vi "Select Worksheet by Name.vi"(2 "error in (no error)":errorcluster, 3 "Worksheet Name":string, 4 "Report Ref In":T1) -> (0 "error out":errorcluster, 1 "Report Ref Out":T1)   [LabVIEW 2013, in "XCel Report Engine.lvlib"]
doc: "Selects a worksheet by name and makes it the active worksheet for subsequent report operations.\n\nThe worksheet name must exactly match an existing worksheet in the open workbook. Worksheet name matching is case-sensitive.\n\nAn error is returned if the name is empty or the worksheet does not exist."
uses:
  XCel Report Engine.lvlib
  C:/Users/m.santucci/Documents/ChatGPT/LV_REPORT_ENGINE/LV/DotNet/XCelReportEngine.dll
  LV/DotNet/XCelReportEngine.dll
  Controls/Report Ref.ctl
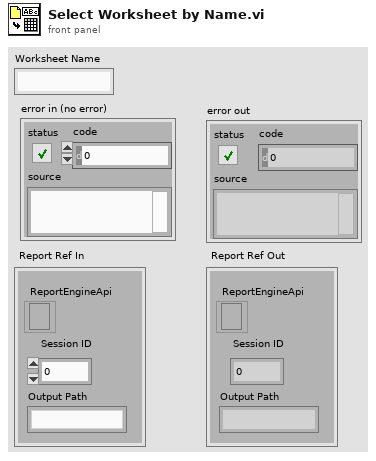
[diagram p1: front panel]
types:
  T1 = typedef "XCel Report Engine.lvlib/Report Ref.ctl" = cluster{"Session ID":i32, "Output Path":string, "ReportEngineApi":refnum<k24>}
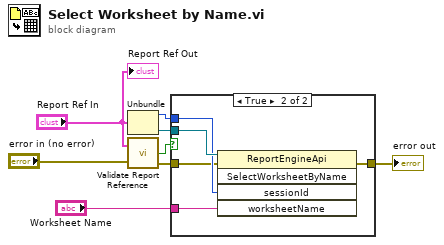
[diagram p0: block diagram]
diagram:
  n1 = Unbundle("Report Ref In") -> ("Session ID"=w7:i32, "ReportEngineApi"=w8:refnum<k24>)  [unwired: 1 out]
  n2 = call "Validate Report Reference.vi"("Report Ref In"="Report Ref In", "error in (no error)"="error in (no error)") -> ("Valid"=w1:bool, "error out"=w2:errorcluster)  [unwired: 1 out]
  n3 = case shown="True" w1 {
    tunnel: w8 -> [_ w14]
    tunnel: w7 -> [_ w13]
    tunnel: "Worksheet Name" -> [_ w12]
    tunnel: [w9 w11] -> w5
    tunnel: w2 -> [w9 w10]
    frame False {
    }
    frame True {
      n4 = invoke class="ReportEngineApi" method="SelectWorksheetByName"(reference=w14, error in=w10, "sessionId"=w13, "worksheetName"=w12) -> (error out=w11:errorcluster)  [unwired: 1 in, 4 out]
    }
  }
  "error out" <- w5
  "Report Ref Out" <- "Report Ref In"
